vi "General - Error Log eFGV.vi"(7 "eFGV States":T1, 8 "error in (no error)":errorcluster, 11 "Error In":string) -> (0 "error out":errorcluster, 2 "Error ref":refnum<user-event>, 3 "Error Out":string)   [LabVIEW 2019]
doc: "event FGV where it will trigger to stop all the process in the program"
uses:
  Controls/eFGV States.ctl
  <vilib>/event_ctls.llb/usereventprio.ctl
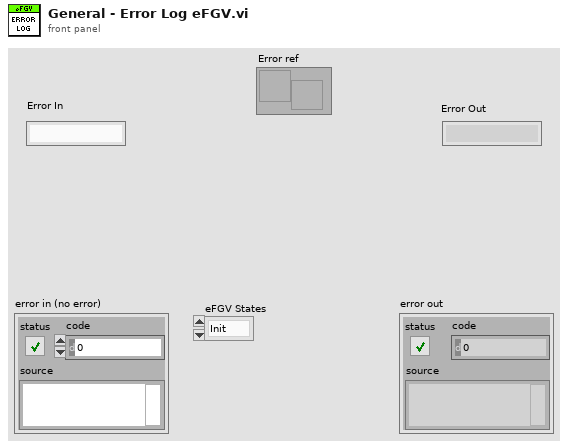
[diagram p1: front panel]
types:
  T1 = typedef "eFGV States.ctl" = enum16{"Init", "Read", "Write", "Exit"}
  T2 = typedef "usereventprio.ctl" = enum32{"high priority", "normal priority"}
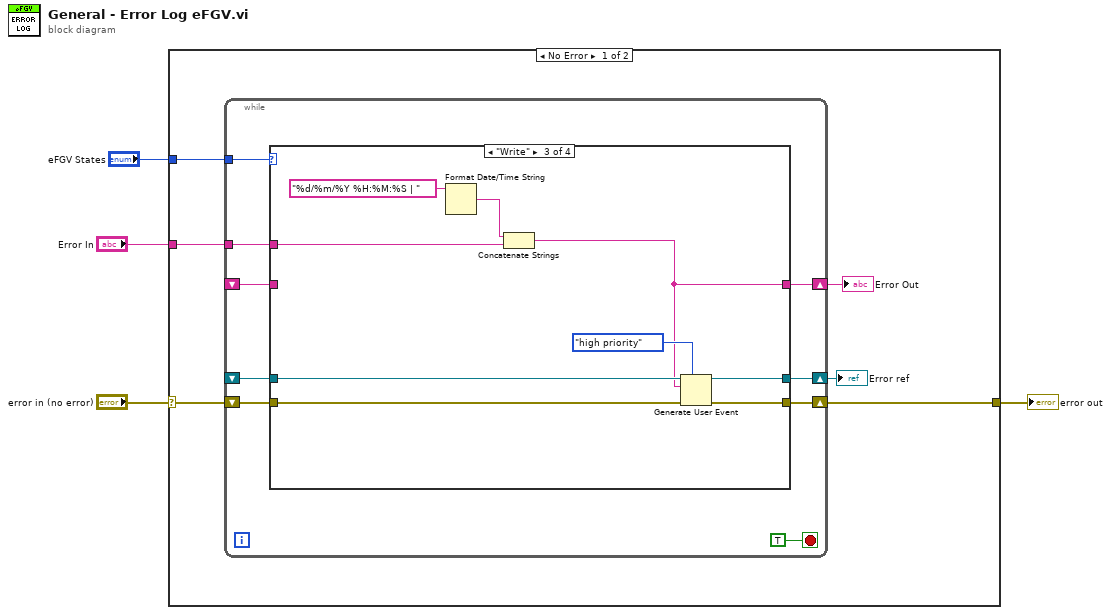
[diagram p0: block diagram]
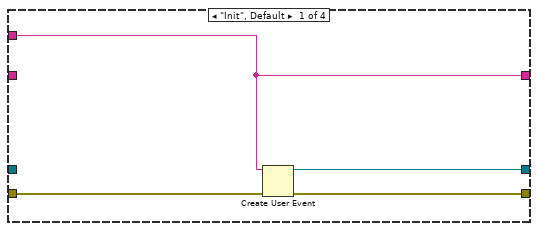
[diagram p2: hidden frame]
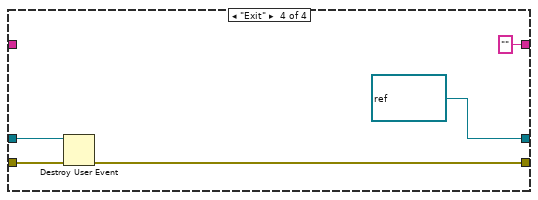
[diagram p4: hidden frame]
diagram:
  n1 = case shown="No Error" "error in (no error)" {
    selector: "error in (no error)" -> [w9 w41]
    tunnel: "eFGV States" -> [w10 _]
    tunnel: "Error In" -> [w8 _]
    tunnel: [w6 w41] -> w1
    frame No Error {
      n2 = while {
        tunnel: w10 -> [w18]
        shift-right: [w15] -> w6
        shift-left: w9 -> [w17]
        tunnel: w8 -> [w16]
        shift-right: [w14] -> w7
        shift-left: _ -> [w13]
        shift-right: [w12] -> w5
        shift-left: _ -> [w11]
        stop <- TRUE stop-if-true
        n3 = case shown="\"Write\"" w18 {
          tunnel: w17 -> [w23 w25 w33 w40]
          tunnel: w16 -> [w21 _ w27 _]
          tunnel: [w22 w25 w34 w38] -> w15
          tunnel: [w21 w26 w28 "" ("Error In")] -> w14
          tunnel: w13 -> [_ w26 _ _]
          tunnel: w11 -> [_ w24 w35 w39]
          tunnel: [w20 w24 w31 refnum<user-event> refnum ("Error In")] -> w12
          frame "Init", Default {
            n4 = Create User Event(user event datatype=w21, error in=w23) -> (user event=w20:refnum<user-event>, error out=w22:errorcluster)
          }
          frame "Read" {
          }
          frame "Write" {
            n5 = Format Date/Time String(time format string (%c)="%d/%m/%Y %H:%M:%S | ") -> (date/time string=w29:string)  [unwired: 2 in]
            n6 = Concatenate Strings(w29, w27) -> (w28:string)
            n7 = Generate User Event(priority (normal)=usereventprio."high priority", user event=w35, event data cluster=w28, error in=w33) -> (user event out=w31:refnum<user-event>, error out=w34:errorcluster)
          }
          frame "Exit" {
            n8 = Destroy User Event(user event=w39, error in=w40) -> (error out=w38:errorcluster)
          }
        }
      }
      "Error Out" <- w7
      "Error ref" <- w5
    }
    frame Error {
    }
  }
  "error out" <- w1
